vi "获取仪器仪表状态.vi"(11 "站号":u16(ring)=3 items=["总磷"=1, "总氮"=2, "氨氮"=3, "CODMn"=21]) -> (3 "工作状态":T1(ring))   [LabVIEW 2016, in "质控单元V4.lvlib"]
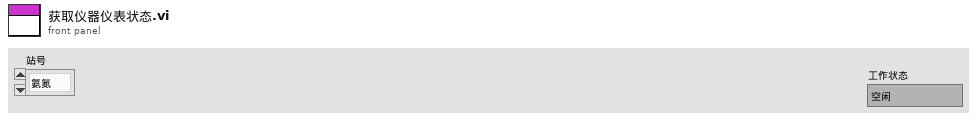
[diagram p1: front panel]
types:
  T1 = enum16{"空闲", "水样测试", "标样核查", "零点核查", "跨度核查", "空白测试", "平行样测试", "加标回收", "空白校准", "标样校准", "初始化（清洗）"}
  T2 = cluster{"系统时间":timestamp, "工作状态":enum16{"空闲", "水样测试", "标样核查", "零点核查", "跨度核查", "空白测试", "平行样测试", "加标回收", "空白校准", "标样校准", "初始化（清洗）"}, "测量模式":enum16{"待机", "连续模式", "周期模式", "定点模式", "受控模式", "手动模式"}, "告警代码":u16, "故障代码":u16, "日志代码":u16, "软件版本":u16}
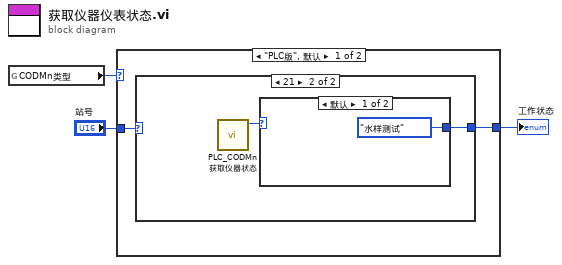
[diagram p0: block diagram]
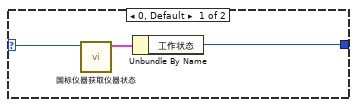
[diagram p2: hidden frame]
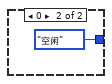
[diagram p3: hidden frame]
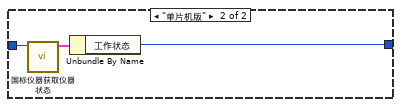
[diagram p4: hidden frame]
diagram:
  n1 = global read "系统交互.vi" "CODMn类型"() -> (w1:enum16{"PLC版", "单片机版"})
  n2 = case shown="\"PLC版\", 默认" w1 {
    tunnel: "站号" -> [w5 w15]
    tunnel: [w4 w14] -> w2
    frame "PLC版", Default {
      n3 = case shown="21" w5 {
        selector: w5 -> [w8 _]
        tunnel: [w6 w9] -> w4
        frame 0, Default {
          n4 = call "国标仪器获取仪器状态.vi"("站号"=w8) -> ("状态告警区"=w7:T2)  [unwired: 9 in, 1 out]
          n5 = Unbundle By Name(w7) -> ("工作状态"=w6:T1)
        }
        frame 21 {
          n6 = call "PLC_CODMn 获取仪器状态.vi"() -> ("CODMn状态"=w10:u16)  [unwired: 11 in]
          n7 = case shown="默认" w10 {
            tunnel: [T1."水样测试" ("工作状态") T1."空闲" ("工作状态")] -> w9
            frame Default {
            }
            frame 0 {
            }
          }
        }
      }
    }
    frame "单片机版" {
      n8 = call "国标仪器获取仪器状态.vi"("站号"=w15) -> ("状态告警区"=w13:T2)  [unwired: 9 in, 1 out]
      n9 = Unbundle By Name(w13) -> ("工作状态"=w14:T1)
    }
  }
  "工作状态" <- w2
